vi "Demo-RandomNumberTest.vi"(11 "YTESTER测试数据":T1 caption="不要修改！") -> (3 "YTESTER结论":T2)   [LabVIEW 2017]
doc: "VIDescription=这是一个DEMO，随机生成合格&不合格结论。"
uses:
  YtCommon.lvlibp/yt`Step StepBaseInput.ctl
  YtCommon.lvlibp/yt`Step StepResult.ctl
  YtCommon.lvlibp/yt`Step TestData.ctl
  YtCommon.lvlibp/yt`Step System Queue.ctl
  YtCommon.lvlibp
panel:
  in  "YTESTER开放参数":T4={"YTESTER_BaseInput"={"isTest"=TRUE, "isSkip"=FALSE, "StepName"="Demo.随机0~1数测试", "OnPass"=enum."Next", "OnFail"=enum."Next", "ReTestNumber"=0.0}, "UpperLimit"=0.75, "LowLimit"=0.25}
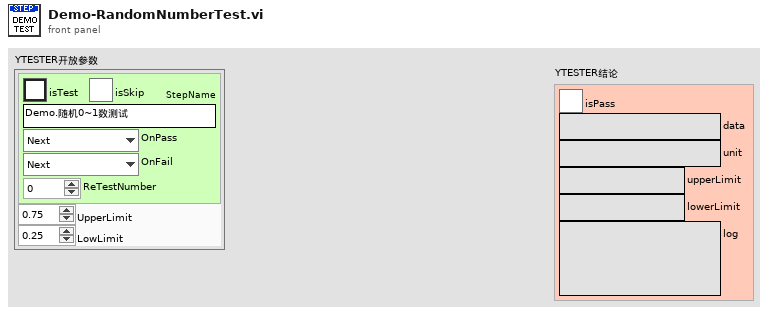
[diagram p1: front panel]
types:
  T1 = typedef "YtCommon.lvlibp/yt`Step TestData.ctl" = cluster{"Socket(From1)":i32, "SN":refnum<notifier>, "StopFlagRef":refnum<notifier>, "YT System Queue":refnum<queue>}
  T2 = typedef "YtCommon.lvlibp/yt`Step StepResult.ctl" = cluster{"isPass":bool, "data":string, "unit":string, "upperLimit":string, "lowerLimit":string, "log":string}
  T3 = typedef "YtCommon.lvlibp/yt`Step StepBaseInput.ctl" = cluster{"isTest":bool, "isSkip":bool, "StepName":string, "OnPass":enum16{"Next", "ToOVER", "Terminate"}, "OnFail":enum16{"Next", "ToOVER", "Terminate"}, "ReTestNumber":dbl}
  T4 = cluster{"YTESTER_BaseInput":T3, "UpperLimit":dbl, "LowLimit":dbl}
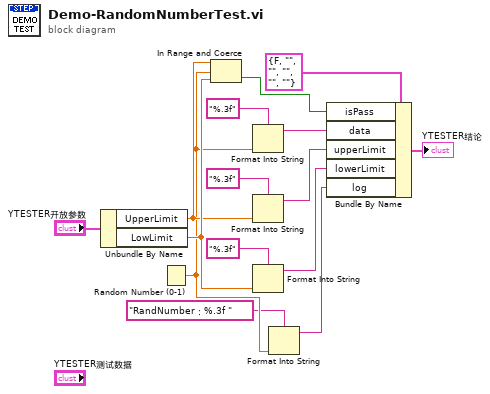
[diagram p0: block diagram]
diagram:
  n1 = Unbundle By Name("YTESTER开放参数") -> ("UpperLimit"=w11:dbl, "LowLimit"=w12:dbl)
  n2 = Random Number (0-1)() -> (number: 0 to 1=w5:dbl)
  n3 = In Range and Coerce(upper limit=w11, x=w5, lower limit=w12) -> (In Range?=w6:bool)  [unwired: 1 out]
  n4 = Format Into String(format string="%.3f", w5) -> (resulting string=w10:string)  [unwired: 2 in, 1 out]
  n5 = Format Into String(format string="%.3f", w11) -> (resulting string=w7:string)  [unwired: 2 in, 1 out]
  n6 = Format Into String(format string="%.3f", w12) -> (resulting string=w8:string)  [unwired: 2 in, 1 out]
  n7 = Format Into String(format string="RandNumber：%.3f ", w5) -> (resulting string=w9:string)  [unwired: 2 in, 1 out]
  n8 = Bundle By Name(cluster=T2 {"isPass"=FALSE, "data"="", "unit"="", "upperLimit"="", "lowerLimit"="", "log"=""} ("Result"), "isPass"=w6, "data"=w10, "upperLimit"=w7, "lowerLimit"=w8, "log"=w9) -> (→"YTESTER结论":T2)
